vi "Host globals (robot acquires video).vi"() -> ()   [LabVIEW 2012]
doc: "Global variables used to define host properties."
panel:
  in  "Safety commands writer name":string="Safety commands writer"
  in  "Video reader endpoint name":string="Video reader"
  in  "Host video timeout":i32=5000
  in  "Host initialization timeout":i32=5000
  in  "Host runtime timeout":i32=1000
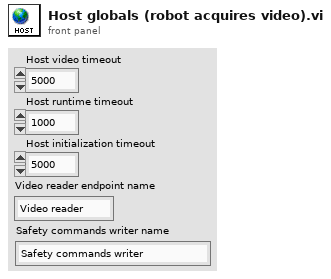
[diagram p1: front panel]
diagram:
